vi "K6514_VISAConfig.vi"(8 "error in (no error)":errorcluster, 11 "VISA resource name":refnum<visa-resource-name>) -> (0 "error out":errorcluster, 3 "reference out":refnum<visa-resource-name>)   [LabVIEW 2024]
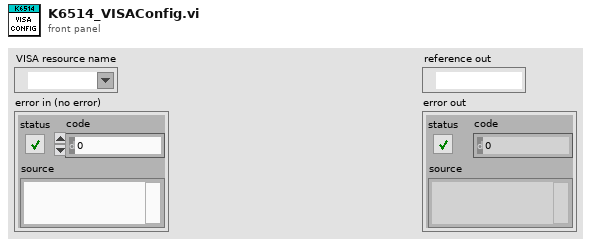
[diagram p1: front panel]
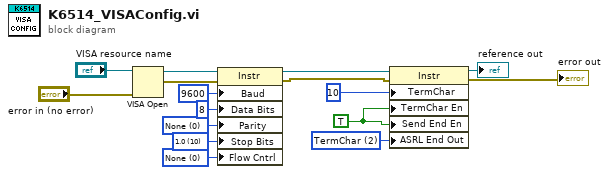
[diagram p0: block diagram]
diagram:
  w6 = u16 0 items=["None", "XON/XOFF", "RTS/CTS", "XON/XOFF & RTS/CTS", "DTR/DSR", "XON/XOFF & DTR/DSR"] ("Serial Settings:Flow Control")
  w7 = u16 10 items=["1.0"=10, "1.5"=15, "2.0"=20] ("Serial Settings:Stop Bits")
  w8 = u16 0 items=["None", "Odd", "Even", "Mark", "Space"] ("Serial Settings:Parity")
  w13 = u16 2 items=["None", "Last Bit", "TermChar", "Break"] ("Serial Settings:End Mode for Writes")
  w15 = TRUE
  n1 = VISA Open(error in (no error)="error in (no error)", VISA resource name="VISA resource name") -> (VISA resource name=w12:refnum<visa-resource-name>, error out=w3:errorcluster)  [unwired: 3 in]
  n2 = property class="Instr"(reference=w12, error in=w3, "Baud"=u32 9600 ("Serial Settings:Baud Rate"), "Data Bits"=u16 8 ("Serial Settings:Data Bits"), "Parity"=w8, "Stop Bits"=w7, "Flow Cntrl"=w6) -> (reference out=w11:refnum<visa-resource-name>, error out=w2:errorcluster)
  n3 = property class="Instr"(reference=w11, error in=w2, "TermChar"=u8 10 ("Termination Character"), "TermChar En"=w15, "Send End En"=w15, "ASRL End Out"=w13) -> (reference out=→"reference out":refnum<visa-resource-name>, error out=→"error out":errorcluster)
